vi "LibXML_GetAttrib.vi"(8 "error in":errorcluster, 9 "index":i32, 10 "attribute":string="name", 11 "XPathObj":u32) -> (0 "error out":errorcluster, 1 "Found":bool, 2 "value":string="y axis", 3 "XPathObj out":u32)   [LabVIEW 2019, in "Tools.lvlib" / "LibXML.lvlib"]
doc: "Get attribute value in XPathObj with name at index input."
uses:
  LibXML.lvlib
  Error Cluster From Error Code_subroutine.vi
  <vilib>/Utility/error.llb/Trim Whitespace.vi
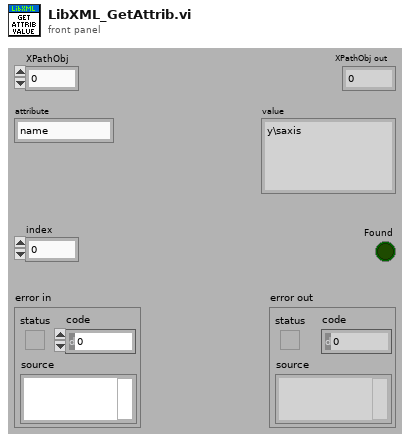
[diagram p1: front panel]
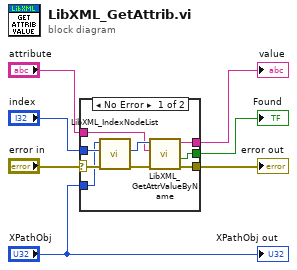
[diagram p0: block diagram]
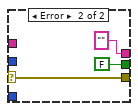
[diagram p2: hidden frame]
diagram:
  n1 = case shown="No Error" "error in" {
    selector: "error in" -> [w15 w19]
    tunnel: [w13 w19] -> w6
    tunnel: [w12 "" ("content")] -> w5
    tunnel: [w11 FALSE ("Found")] -> w4
    tunnel: "index" -> [w10 _]
    tunnel: "XPathObj" -> [w9 _]
    tunnel: "attribute" -> [w8 _]
    frame No Error {
      n2 = call "LibXML_IndexNodeList.vi"("error in"=w15, "index"=w10, "XPathObj"=w9) -> ("error out"=w14:errorcluster, "NodePtr"=w16:u32)  [unwired: 6 in, 1 out]
      n3 = call "LibXML_GetAttrValueByName.vi"("error in"=w14, "attribute"=w8, "node"=w16) -> ("error out"=w13:errorcluster, "Found"=w11:bool, "lvstring"=w12:string)  [unwired: 6 in]
    }
    frame Error {
    }
  }
  "error out" <- w6
  "value" <- w5
  "Found" <- w4
  "XPathObj out" <- "XPathObj"
